vi "SEQ Release Queue.vi"(8 "error in":errorcluster) -> (0 "error out":errorcluster)   [LabVIEW 2019, in "Andor.lvlib"]
uses:
  Andor.lvlib
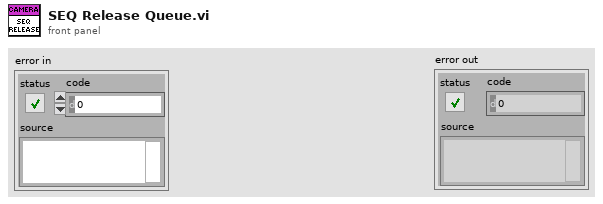
[diagram p1: front panel]
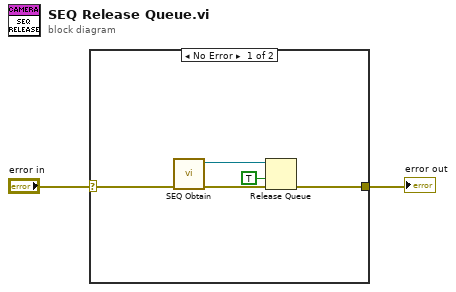
[diagram p0: block diagram]
diagram:
  n1 = case shown="No Error" "error in" {
    selector: "error in" -> [w5 w8]
    tunnel: [w6 w8] -> w1
    frame No Error {
      n2 = call "SEQ Obtain.vi"("error in"=w5) -> ("error out"=w4:errorcluster, "queue out"=w3:refnum<queue>)  [unwired: 9 in]
      n3 = Release Queue(queue=w3, force destroy? (F)=TRUE, error in (no error)=w4) -> (error out=w6:errorcluster)  [unwired: 2 out]
    }
    frame Error {
    }
  }
  "error out" <- w1
